vi "SPTI Write10 Command.vi"(7 "Data to be Written":u8[](array[numeric]), 8 "error in (no error)":errorcluster, 9 "Block Size (512)":u32=512, 10 "Nr Blocks":u32, 11 "Start LBA":u32 format="%08x") -> (0 "error out":errorcluster, 3 "Read Data":u8[](array[numeric]) format="%02x")   [LabVIEW 2014]
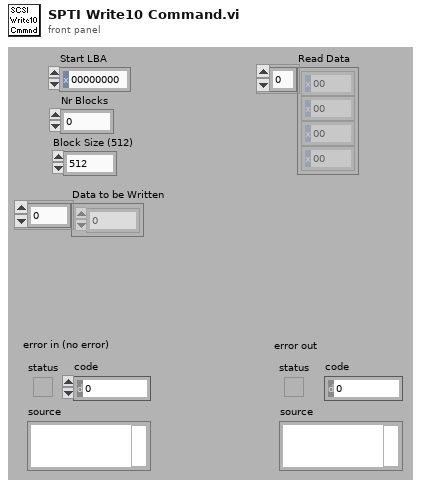
[diagram p1: front panel]
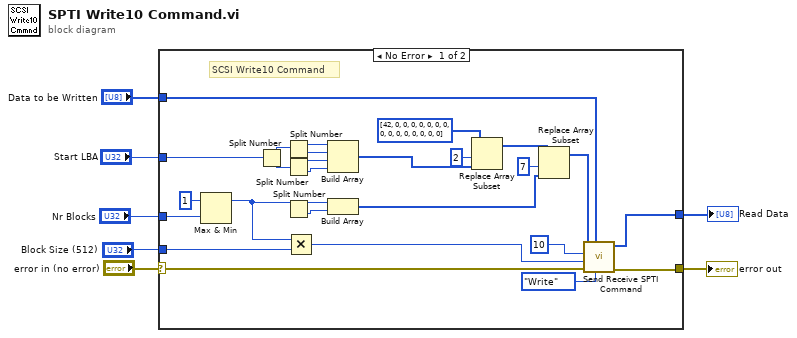
[diagram p0: block diagram]
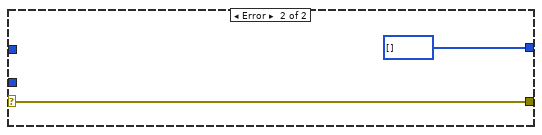
[diagram p2: hidden frame]
diagram:
  n1 = case shown="No Error" "error in (no error)" {
    selector: "error in (no error)" -> [w34 w36]
    tunnel: [w31 w36] -> w6
    tunnel: "Start LBA" -> [w30 _]
    tunnel: "Nr Blocks" -> [w20 _]
    tunnel: "Block Size (512)" -> [w21 _]
    tunnel: [w16 u8[] [] ("Received Data")] -> w2
    tunnel: "Data to be Written" -> [w8 _]
    frame No Error {
      # "SCSI Write10 Command"
      n2 = Max & Min(x=u32 1, y=w20) -> (max(x,y)=w11:u32)  [unwired: 1 out]
      n3 = Split Number(x=w30) -> (hi(x)=w29:u16, lo(x)=w28:u16)
      n4 = Split Number(x=w29) -> (hi(x)=w27:u8, lo(x)=w26:u8)
      n5 = Split Number(x=w28) -> (hi(x)=w25:u8, lo(x)=w24:u8)
      n6 = Split Number(x=w11) -> (hi(x)=w22:u16, lo(x)=w23:u16)
      n7 = Multiply(x=w11, y=w21) -> (x*y=w19:u32)
      n8 = Build Array(w27, w26, w25, w24) -> (w14:u8[])
      n9 = Build Array(w22, w23) -> (w10:u16[])
      n10 = Replace Array Subset(array=u8[] [42, 0, 0, 0, 0, 0, 0, 0, 0, 0, 0, 0, 0, 0, 0, 0] ("Command Data Block"), new element=w14, index=2) -> (w13:u8[])
      n11 = Replace Array Subset(array=w13, new element=w10, index=7) -> (w9:u8[])
      n12 = call "Send Receive SPTI Command.vi"("read/write"=enum16{"Read", "Write"}."Write", "Data to be Written"=w8, "error in (no error)"=w34, "Expected Nr Response Bytes"=w19, "Valid CDB bytes"=u8 10, "Command Data Block"=w9) -> ("error out"=w31:errorcluster, "Received Data"=w16:u8[])  [unwired: 4 in]
    }
    frame Error {
    }
  }
  "error out" <- w6
  "Read Data" <- w2
